vi "Read Configuration.vi"(8 "error in (no error)":errorcluster, 11 "H-Intfc in":refnum<class "REST Interface.lvclass">) -> (0 "error out":errorcluster, 2 "Configuration.lvlibp:Configuration.lvclass":refnum<class "Configuration.lvclass">, 3 "H-Intfc out":refnum<class "REST Interface.lvclass">)   [LabVIEW 2018, in "REST Interface.lvlib" / "REST Interface.lvclass"]
uses:
  REST Interface.lvclass
  PPLs/Configuration/Configuration.lvlibp/Configuration.lvclass
  REST Interface.lvclass/REST Interface.ctl
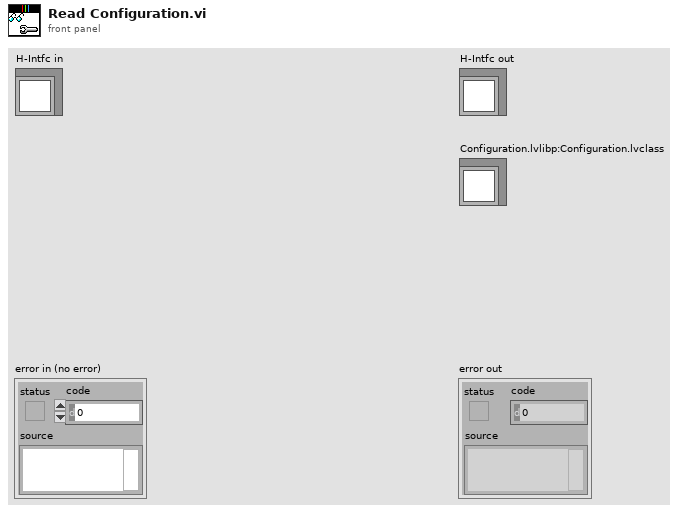
[diagram p1: front panel]
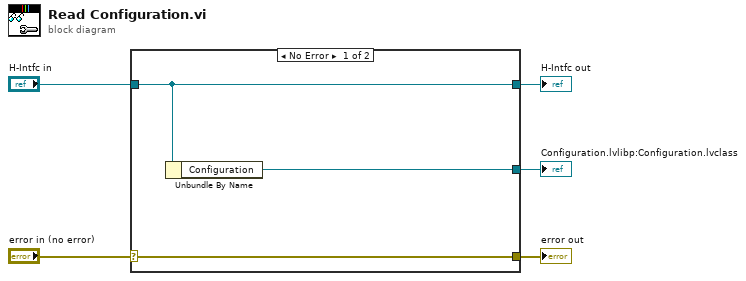
[diagram p0: block diagram]
diagram:
  n1 = case shown="No Error" "error in (no error)" {
    selector: "error in (no error)" -> [w8 w9]
    tunnel: [w8 w9] -> w4
    tunnel: [w7 w10] -> w2
    tunnel: "H-Intfc in" -> [w7 w10]
    tunnel: [w6 _] -> w1
    frame No Error {
      n2 = Unbundle By Name(w7) -> ("Configuration"=w6:refnum<class "Configuration.lvclass">)
    }
    frame Error {
    }
  }
  "error out" <- w4
  "H-Intfc out" <- w2
  "Configuration.lvlibp:Configuration.lvclass" <- w1
